vi "GetButtonsStates (SubVI).vi"(7 "LINX Resource":T1, 8 "reference":refnum<vi>) -> ()   [LabVIEW 2014]
uses:
  <vilib>/MakerHub/LINX/Private/Type Defs/LINX Ref.ctl
  <vilib>/MakerHub/LINX/Private/Type Defs/Platform.ctl
  <vilib>/MakerHub/LINX/Private/Type Defs/Interface.ctl
  <vilib>/MakerHub/LINX/Private/Device/Type Defs/LINX Device Config.ctl
  <vilib>/MakerHub/LINX/Private/Device/Type Defs/TCP Config.ctl
  <vilib>/MakerHub/LINX/Private/Device/Type Defs/Channels.ctl
  <vilib>/MakerHub/LINX/Public/Peripherals/Digital/Digital Read 1 Chan.vi
  <vilib>/MakerHub/LINX/Public/Peripherals/Digital/Digital Read N Chans.vi
  <vilib>/MakerHub/LINX/Private/Local IO/LinxDigitalRead.vi
  <vilib>/MakerHub/LINX/Public/Utilities/Check Channel.vi
  <vilib>/MakerHub/LINX/Private/Local IO/Handle Errors.vi
  <vilib>/MakerHub/LINX/Private/Utilties/Generate Error.vi
  <vilib>/MakerHub/LINX/LMH-LINX.lvlib
  <vilib>/MakerHub/LINX/Private/Device/Device.lvlib
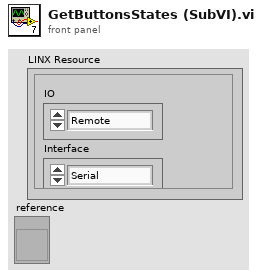
[diagram p1: front panel]
types:
  T1 = typedef "LMH-LINX.lvlib/LINX Ref.ctl" = cluster{"IO":T2, "Interface":T3, "LINX Device Config":T4}
  T2 = typedef "LMH-LINX.lvlib/Platform.ctl" = enum16{"Remote", "Local"}
  T3 = typedef "LMH-LINX.lvlib/Interface.ctl" = enum16{"Serial", "TCP"}
  T4 = typedef "LMH-LINX.lvlib/Device.lvlib/LINX Device Config.ctl" = cluster{"Interface":T3, "COM Port":refnum<visa-resource-name>, "TCP Configuration":T5, "Device Family":u8, "Device ID":u8, "Device Name":string, "TCP Ref":refnum<k5>, "Channels":T6}
  T5 = typedef "LMH-LINX.lvlib/Device.lvlib/TCP Config.ctl" = cluster{"IP Address":string, "Port":u16}
  T6 = typedef "LMH-LINX.lvlib/Channels.ctl" = cluster{"DI":u8[], "DO":u8[], "AI":u8[], "AO":u8[], "PWM":u8[], "QE":u8[], "UART":u8[], "I2C 2":u8[], "SPI":u8[], "CAN":u8[], "Servo":u8[], "AI Ref (V)":dbl, "AI Resolution (Bits)":u8, "AO Ref (V)":dbl, "AO Resolution (Bits)":u8}
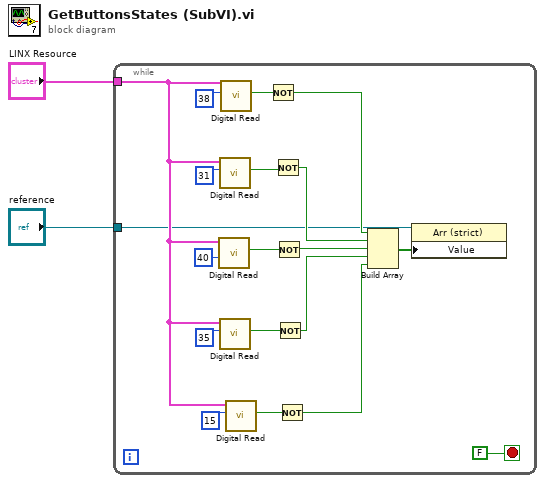
[diagram p0: block diagram]
diagram:
  n1 = while {
    tunnel: "LINX Resource" -> [w11]
    tunnel: "reference" -> [w3]
    stop <- FALSE stop-if-true
    n2 = call-poly <vilib>:"Digital Read.vi"("DI Channel"=40, "LINX Resource"=w11) -> ("DI Value"=w14:bool)  [unwired: 7 in, 2 out]
    n3 = call-poly <vilib>:"Digital Read.vi"("DI Channel"=31, "LINX Resource"=w11) -> ("DI Value"=w15:bool)  [unwired: 7 in, 2 out]
    n4 = call-poly <vilib>:"Digital Read.vi"("DI Channel"=35, "LINX Resource"=w11) -> ("DI Value"=w13:bool)  [unwired: 7 in, 2 out]
    n5 = call-poly <vilib>:"Digital Read.vi"("DI Channel"=38, "LINX Resource"=w11) -> ("DI Value"=w16:bool)  [unwired: 7 in, 2 out]
    n6 = call-poly <vilib>:"Digital Read.vi"("DI Channel"=15, "LINX Resource"=w11) -> ("DI Value"=w10:bool)  [unwired: 7 in, 2 out]
    n7 = Not(x=w16) -> (.not. x?=w5:bool)
    n8 = Not(x=w15) -> (.not. x?=w9:bool)
    n9 = Not(x=w14) -> (.not. x?=w8:bool)
    n10 = Not(x=w13) -> (.not. x?=w6:bool)
    n11 = Not(x=w10) -> (.not. x?=w7:bool)
    n12 = Build Array(w5, w9, w8, w6, w7) -> (w4:bool[])
    n13 = property class="Arr (strict)"(reference=w3, "Value"=w4) -> ()  [unwired: 1 in, 2 out]
  }
